vi "close&save.vi"(8 "error in":errorcluster, 11 "input cluster":T1={"Users"=[{"Name"="John", "Surname"="Doe", "Cash"=2000, "PIN"=""}, {"Name"="Jennifer", "Surname"="Rodriguez", "Cash"=1500, "PIN"=""}, {"Name"="Bryan", "Surname"="Smith", "Cash"=800, "PIN"=""}, {"Name"="Julie", "Surname"="Ramirez", "Cash"=900, "PIN"=""}], "Customer"={"Name"="", "Surname"="", "Cash"=0, "PIN"=""}, "Message"="", "Right Menu"={"RFS String"="", "RFS String 2"="", "RFS String 3"=""}, "Left Menu"={"RFS String"="", "RFS String 2"="", "RFS String 3"=""}}) -> (0 "error out":errorcluster)   [LabVIEW 2015]
uses:
  Users Data.ctl
  Controls/User data.ctl
  <vilib>/Utility/file.llb/Write Delimited Spreadsheet (string).vi
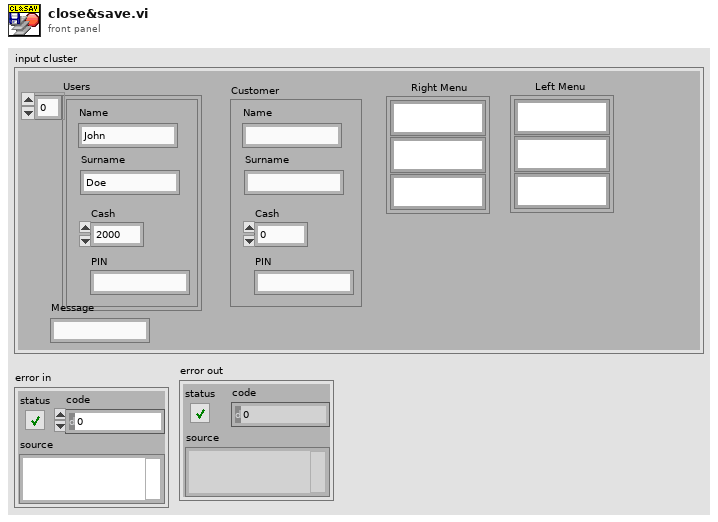
[diagram p1: front panel]
types:
  T1 = typedef "Users Data.ctl" = cluster{"Users":T2[], "Customer":T2, "Message":string, "Right Menu":cluster{"RFS String":string, "RFS String 2":string, "RFS String 3":string}, "Left Menu":cluster{"RFS String":string, "RFS String 2":string, "RFS String 3":string}}
  T2 = typedef "User data.ctl" = cluster{"Name":string, "Surname":string, "Cash":i32, "PIN":string}
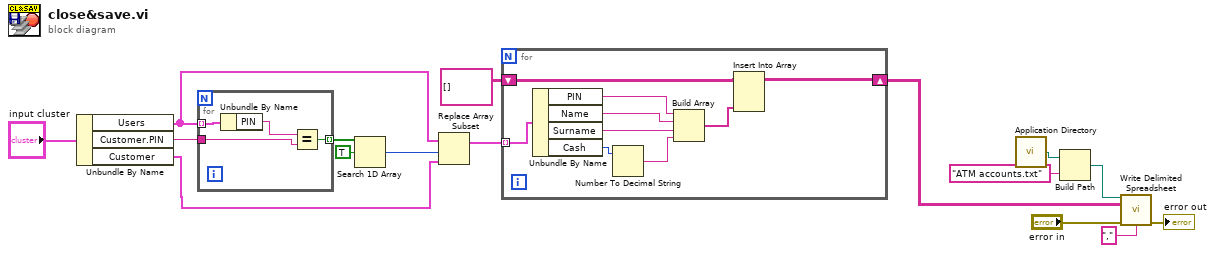
[diagram p0: block diagram]
diagram:
  n1 = Unbundle By Name("input cluster") -> ("Users"=w6:T2[], "Customer.PIN"=w2:string, "Customer"=w7:T2)
  n2 = for {
    tunnel: w6 -> [w20] mode=indexing
    tunnel: w2 -> [w18]
    tunnel: [w17] -> w3 mode=indexing
    n3 = Unbundle By Name(w20) -> ("PIN"=w19:string)
    n4 = Equal?(x=w19, y=w18) -> (x = y?=w17:bool)
  }
  n5 = Search 1D Array(1D array=w3, element=TRUE) -> (index of element=w5:i32)  [unwired: 1 in]
  n6 = Replace Array Subset(array=w6, new element=w7, index=w5) -> (w8:T2[])
  n7 = for {
    tunnel: w8 -> [w29] mode=indexing
    shift-right: [w23] -> w13
    shift-left: string[][] [] -> [w22]
    n8 = Unbundle By Name(w29) -> ("PIN"=w27:string, "Name"=w26:string, "Surname"=w25:string, "Cash"=w28:i32)
    n9 = Number To Decimal String(number=w28) -> (decimal integer string=w24:string)  [unwired: 1 in]
    n10 = Build Array(w27, w26, w25, w24) -> (w21:string[])
    n11 = Insert Into Array(array=w22, new element=w21) -> (w23:string[][])  [unwired: 2 in]
  }
  n12 = call <vilib>:"Application Directory.vi"() -> ("Application Directory"=w11:path)
  n13 = Build Path(base path=w11, name or relative path="ATM accounts.txt") -> (appended path=w12:path)
  n14 = call-poly <vilib>:"Write Delimited Spreadsheet.vi"("file path (dialog if empty)"=w12, "2D data"=w13, "error in (no error)"="error in", "delimiter (\\t)"="," ("delimiter (\\t)")) -> ("error out"=→"error out":errorcluster)  [unwired: 10 in, 1 out]
